vi "ROS_Master_removePubSub.vi"(2 "Direction":enum16{"Publisher", "Subscriber"}(ring)=enum."Subscriber", 3 "PubSub":T5, 4 "ROS_Master in":T1) -> (0 "error out":errorcluster, 1 "ROS_Master our":T1)   [LabVIEW 2015]
doc: "Unregisters a publisher or subscriber with the master and updates list of publishers and subscribers to reflect change"
uses:
  ROS_Master.ctl
  ROS_Topic.ctl
  ROS_Node.ctl
  ROS_Service.ctl
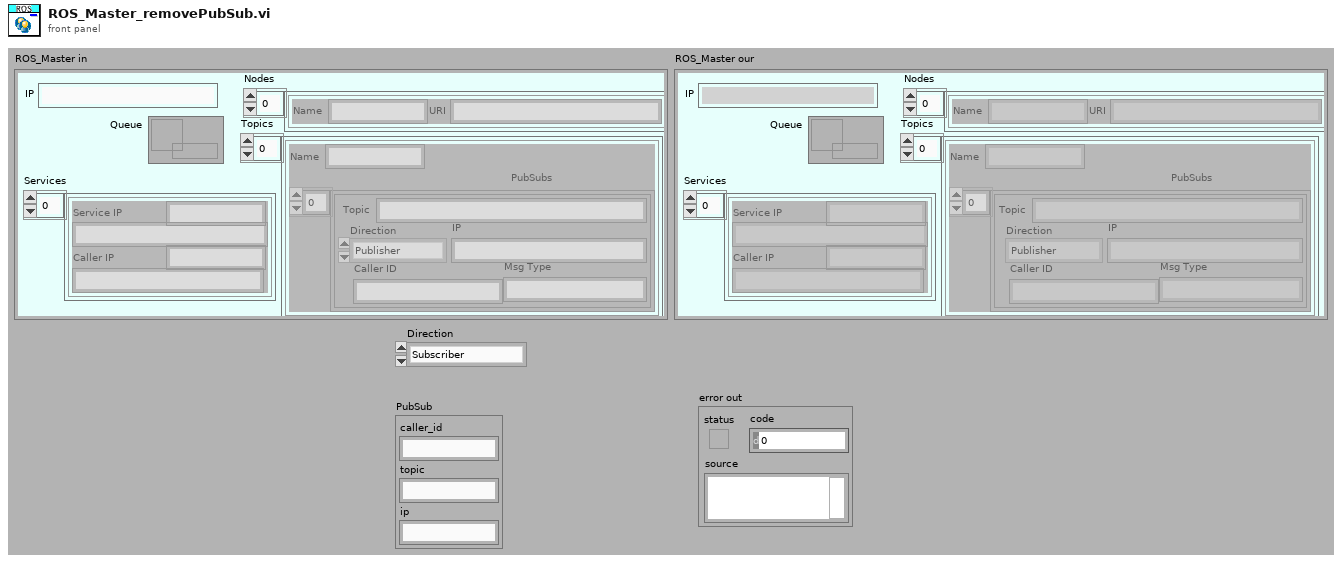
[diagram p1: front panel]
types:
  T1 = typedef "ROS_Master.ctl" = cluster{"IP":string, "Topics":cluster{"Name":string, "PubSubs":T2[]}[], "Nodes":T3[], "Services":T4[], "Queue":refnum<queue>}
  T2 = typedef "ROS_Topic.ctl" = cluster{"Caller ID":string, "IP":string, "Msg Type":string, "Direction":enum16{"Publisher", "Subscriber"}, "Topic":string}
  T3 = typedef "ROS_Node.ctl" = cluster{"Name":string, "URI":string}
  T4 = typedef "ROS_Service.ctl" = cluster{"Service":string, "Service IP":string, "Caller IP":string, "Caller ID":string}
  T5 = cluster{"caller_id":string, "topic":string, "ip":string}
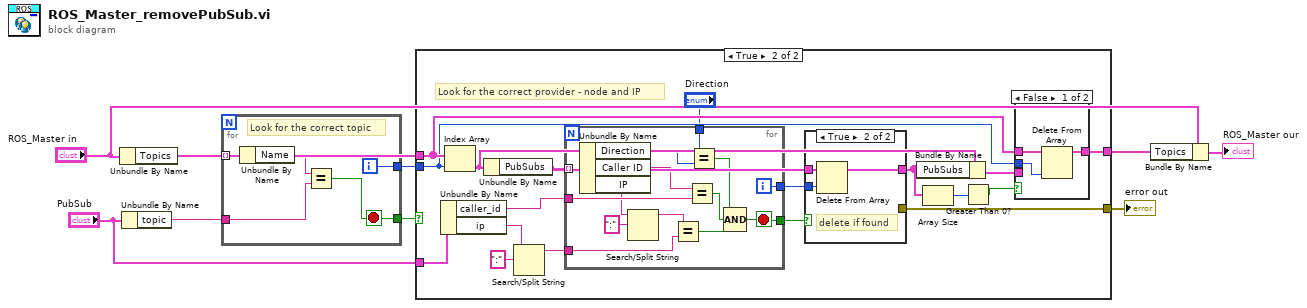
[diagram p0: block diagram]
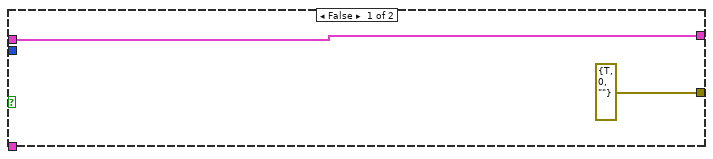
[diagram p2: hidden frame]
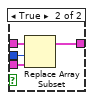
[diagram p3: hidden frame]
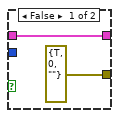
[diagram p4: hidden frame]
diagram:
  n1 = Unbundle By Name("ROS_Master in") -> ("Topics"=w8:cluster{"Name":string, "PubSubs":T2[]}[])
  n2 = Unbundle By Name("PubSub") -> ("topic"=w9:string)
  n3 = for {
    tunnel: w8 -> [w14] mode=indexing
    tunnel: w9 -> [w12]
    tunnel: [w11] -> w7
    tunnel: [w10] -> w5
    i -> [w11]
    stop <- w10 stop-if-true
    # "Look for the correct topic"
    n4 = Unbundle By Name(w14) -> ("Name"=w13:string)
    n5 = Equal?(x=w13, y=w12) -> (x = y?=w10:bool)
  }
  n6 = case shown="True" w5 {
    tunnel: w8 -> [w16 w28]
    tunnel: w7 -> [_ w25]
    tunnel: "PubSub" -> [_ w34]
    tunnel: [w16 w26] -> w4
    tunnel: [errorcluster {"status"=TRUE, "code"=0, "source"=""} ("error constant") w24] -> w3
    frame False {
    }
    frame True {
      # "Look for the correct provider - node and IP"
      n7 = Unbundle By Name(w34) -> ("caller_id"=w33:string, "ip"=w21:string)
      n8 = Index Array(array=w28, index=w25) -> (element=w29:cluster{"Name":string, "PubSubs":T2[]})
      n9 = Unbundle By Name(w29) -> ("PubSubs"=w32:T2[])
      n10 = Search/Split String(string=w21, search string/char (-)=":") -> (substring before match=w20:string)  [unwired: 1 in, 2 out]
      n11 = for {
        tunnel: w32 -> [w60] mode=indexing
        tunnel: w33 -> [w58]
        tunnel: [w54] -> w31
        tunnel: [w57] -> w30
        tunnel: "Direction" -> [w52]
        tunnel: w20 -> [w48]
        i -> [w57]
        stop <- w54 stop-if-true
        n12 = Unbundle By Name(w60) -> ("Direction"=w53:enum16{"Publisher", "Subscriber"}, "Caller ID"=w59:string, "IP"=w50:string)
        n13 = Search/Split String(string=w50, search string/char (-)=":") -> (substring before match=w49:string)  [unwired: 1 in, 2 out]
        n14 = Equal?(x=w49, y=w48) -> (x = y?=w47:bool)
        n15 = Equal?(x=w59, y=w58) -> (x = y?=w56:bool)
        n16 = Equal?(x=w52, y=w53) -> (x = y?=w55:bool)
        n17 = Compound Arithmetic op=AND(w55, w56, w47) -> (w54:bool)
      }
      n18 = case shown="True" w31 {
        tunnel: w32 -> [w43 w46]
        tunnel: w30 -> [_ w45]
        tunnel: [w43 w44] -> w19
        tunnel: [errorcluster {"status"=TRUE, "code"=0, "source"=""} ("error constant") _] -> w24
        frame False {
        }
        frame True {
          # "delete if found"
          n19 = Delete From Array(array=w46, index=w45) -> (array with subset deleted=w44:T2[])  [unwired: 1 in, 1 out]
        }
      }
      n20 = Bundle By Name(cluster=w29, "PubSubs"=w19) -> (w27:cluster{"Name":string, "PubSubs":T2[]})
      n21 = Array Size(array=w19) -> (size(s)=w18:i32)
      n22 = Greater Than 0?(x=w18) -> (x > 0?=w17:bool)
      n23 = case shown="False" w17 {
        tunnel: w28 -> [w37 w41]
        tunnel: w27 -> [_ w40]
        tunnel: [w36 w39] -> w26
        tunnel: w25 -> [w35 w38]
        frame False {
          n24 = Delete From Array(array=w37, index=w35) -> (array with subset deleted=w36:cluster{"Name":string, "PubSubs":T2[]}[])  [unwired: 1 in, 1 out]
        }
        frame True {
          n25 = Replace Array Subset(array=w41, new element=w40, index=w38) -> (w39:cluster{"Name":string, "PubSubs":T2[]}[])
        }
      }
    }
  }
  "error out" <- w3
  n26 = Bundle By Name(cluster="ROS_Master in", "Topics"=w4) -> (→"ROS_Master our":T1)
